vi "MGI Hex Str to U8 Data.vi"(1 "HEX String (0-9,A-F)":string) -> (0 "u8 Data[]":u8[](array[numeric]) format="%.0x")   [LabVIEW 2020]
doc: "Convert the Hex String containing 0-9 and A-F to an array of bytes.\nNOTE: This VI does not handle lower case a-f.\n\nAuthored by Shawn Walpole\nsupport@mooregoodideas.com\nwww.mooregoodideas.com\n\nCopyright (c) 2010, Moore Good Ideas, Inc.\n\nAll rights reserved.\n\nRedistribution and use in source and binary forms, with or without modification, are permitted provided that the following conditions are met:\n\n * Redistributions of source code must retain the above copyright notice, this list of conditions and the following disclaimer.\n * Redistributions in binary form must reproduce the above copyright notice, this list of conditions and the following disclaimer in the documentation and/or other materials provided with the distribution.\n * Neither the name of Moore Good Ideas, Inc. nor the names of its contributors may be used to endorse or promote products derived from this software without specific prior written permission.\n\nTHIS SOFTWARE IS PROVIDED BY THE COPYRIGHT HOLDERS AND CONTRIBUTORS \"AS IS\" AND ANY EXPRESS OR IMPLIED WARRANTIES, INCLUDING, BUT NOT LIMITED TO, THE IMPLIED WARRANTIES OF MERCHANTABILITY AND FITNESS FOR A PARTICULAR PURPOSE ARE DISCLAIMED. IN NO EVENT SHALL THE COPYRIGHT OWNER OR CONTRIBUTORS BE LIABLE FOR ANY DIRECT, INDIRECT, INCIDENTAL, SPECIAL, EXEMPLARY, OR CONSEQUENTIAL DAMAGES (INCLUDING, BUT NOT LIMITED TO, PROCUREMENT OF SUBSTITUTE GOODS OR SERVICES; LOSS OF USE, DATA, OR PROFITS; OR BUSINESS INTERRUPTION) HOWEVER CAUSED AND ON ANY THEORY OF LIABILITY, WHETHER IN CONTRACT, STRICT LIABILITY, OR TORT (INCLUDING NEGLIGENCE OR OTHERWISE) ARISING IN ANY WAY OUT OF THE USE OF THIS SOFTWARE, EVEN IF ADVISED OF THE POSSIBILITY OF SUCH DAMAGE."
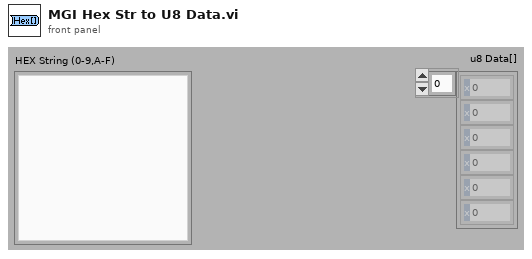
[diagram p1: front panel]
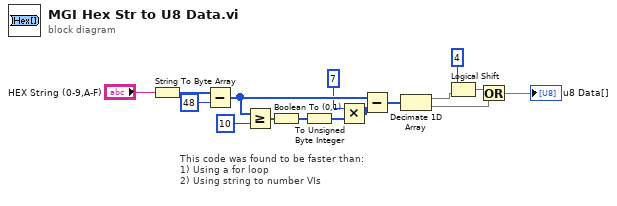
[diagram p0: block diagram]
diagram:
  # "This code was found to be faster than:\n1) Using a for loop\n2) Using string to number VIs"
  n1 = String To Byte Array(string="HEX String (0-9,A-F)") -> (unsigned byte array=w1:u8[])
  n2 = Subtract(x=w1, y=u8 48) -> (x-y=w14:u8[])
  n3 = Greater Or Equal?(x=w14, y=u8 10) -> (x >= y?=w11:bool[])
  n4 = Boolean To (0,1)(Boolean=w11) -> (0, 1=w9:i16[])
  n5 = To Unsigned Byte Integer(number=w9) -> (unsigned 8bit integer=w12:u8[])
  n6 = Multiply(x=u8 7, y=w12) -> (x*y=w13:u8[])
  n7 = Subtract(x=w14, y=w13) -> (x-y=w3:u8[])
  n8 = Decimate 1D Array(w3) -> (w4:u8[], w2:u8[])
  n9 = Logical Shift(y=i8 4, x=w4) -> (x << y=w15:u8[])
  n10 = Or(x=w15, y=w2) -> (x .or. y?=→"u8 Data[]":u8[])
